vi "PasteSafe.vi"(4 "ModeCol Index":i32=2, 5 "Layout Ref":refnum<vi>, 6 "Cell Start":T1, 7 "Table History ref":refnum<vi>, 8 "error in (no error)":errorcluster, 9 "Table CtlRef In":refnum<vi>, 10 "Clipboard (clipped)":string[][](array[string]), 11 "Col Array Ref in":refnum<vi>) -> (0 "error out":errorcluster, 1 "Table CtlRef Out":refnum<vi>, 3 "Col Array Ref out":refnum<vi>)   [LabVIEW 2013]
doc: "Paste input \"Clipboard (clipped)\" into Table beginning at Cell Start. This function won't overwrite a disabled cell, only checks Mode column if necessary, and takes care of reformatting table. Also, the previous table value is pushed to Table History (if \"Table History ref\" is wired).\n\nThis VI is read-only w.r.t column array."
uses:
  <vilib>/Utility/miscctls.llb/LVRowAndColumnTypeDef.ctl
  TypeDefs/TableHistory.ctl
  TypeDefs/TableArray.ctl
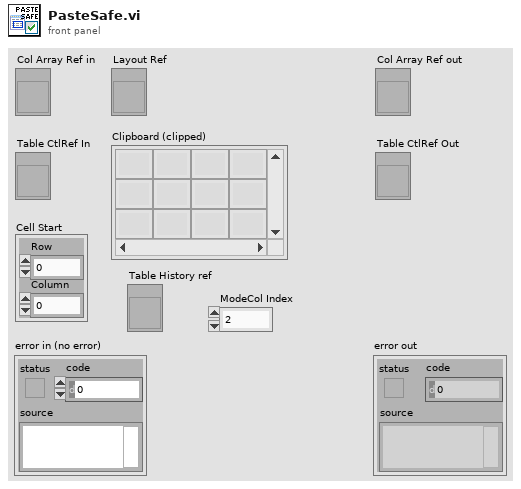
[diagram p1: front panel]
types:
  T1 = typedef "LVRowAndColumnTypeDef.ctl" = cluster{"Row":i32, "Column":i32}
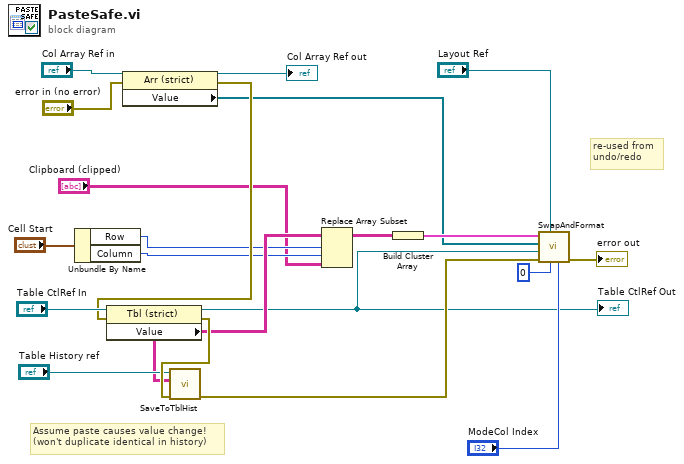
[diagram p0: block diagram]
diagram:
  # "re-used from\nundo/redo"
  # "Assume paste causes value change!\n(won't duplicate identical in history)"
  n1 = Unbundle By Name("Cell Start") -> ("Row"=w12:i32, "Column"=w2:i32)
  n2 = property class="Arr (strict)"(reference="Col Array Ref in", error in="error in (no error)") -> (reference out=→"Col Array Ref out":refnum<vi>, error out=w16:errorcluster, "Value"=w6:refnum<class "Column.lvclass">[])
  n3 = property class="Tbl (strict)"(reference="Table CtlRef In", error in=w16) -> (reference out=w4:refnum<vi>, error out=w15:errorcluster, "Value"=w13:string[][])
  "Table CtlRef Out" <- w4
  n4 = call "SaveToTblHist.vi"("error in (no error)"=w15, "OldTable (reset)"=w13, "Table History ref"="Table History ref") -> ("error out"=w11:errorcluster)  [unwired: 8 in]
  n5 = Replace Array Subset(array=w13, new element="Clipboard (clipped)", index (row)=w12, index (col)=w2) -> (w8:string[][])
  n6 = Build Cluster Array(w8) -> (w7:cluster{"Value":string[][]}[])
  n7 = call "SwapAndFormat.vi"("Mode Index"="ModeCol Index", "Undo pointer"=0, "Layout Ref"="Layout Ref", "error in (no error)"=w11, "Table CtlRef In"=w4, "Col Array in"=w6, "OldTable Array in"=w7) -> ("error out"=→"error out":errorcluster)  [unwired: 3 in, 1 out]
